vi "ITC Send Command.vi"(1 "Command":string) -> (0 "Response":string)   [LabVIEW 2009]
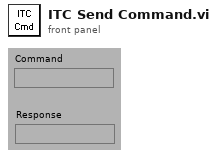
[diagram p1: front panel]
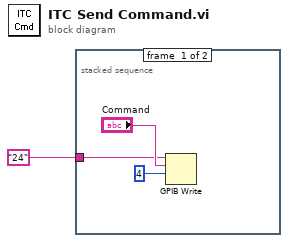
[diagram p0: block diagram]
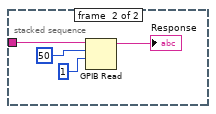
[diagram p2: hidden frame]
diagram:
  n1 = stacked-sequence {
    tunnel: "24" -> [w2 w6]
    frame #0 {
      n2 = GPIB Write(0:w2, 1:"Command", 2:i16 4 ("mode (0)")) -> ()  [unwired: 2 in, 2 out]
    }
    frame #1 {
      n3 = GPIB Read(0:w6, 1:50 ("byte count"), 2:i16 1 ("mode (0)")) -> (5:→"Response":string)  [unwired: 2 in, 2 out]
    }
  }
